vi "stripCRLF.vi"(10 "CRLF terminated String":string) -> (2 "unterminated String":string)   [LabVIEW 2014]
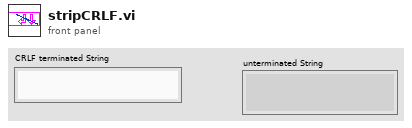
[diagram p1: front panel]
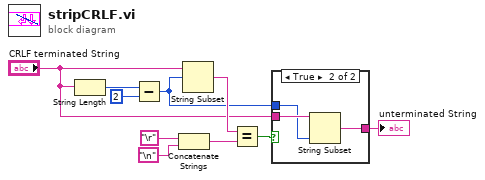
[diagram p0: block diagram]
diagram:
  n1 = String Length(string="CRLF terminated String") -> (length=w10:i32)
  n2 = Subtract(x=w10, y=2) -> (x-y=w2:i32)
  n3 = Concatenate Strings("\r", "\n") -> (w6:string)
  n4 = String Subset(string="CRLF terminated String", offset (0)=w2) -> (substring=w5:string)  [unwired: 1 in]
  n5 = Equal?(x=w5, y=w6) -> (x = y?=w4:bool)
  n6 = case shown="True" w4 {
    tunnel: "CRLF terminated String" -> [w11 w14]
    tunnel: w2 -> [_ w13]
    tunnel: [w11 w12] -> w1
    frame False {
    }
    frame True {
      n7 = String Subset(string=w14, length (rest)=w13) -> (substring=w12:string)  [unwired: 1 in]
    }
  }
  "unterminated String" <- w1
